vi "Parameter Set Write Single.vi"(8 "error in":errorcluster, 9 "Channel Index":i32, 10 "Parameter Set STS":i32, 11 "Parameter Set in":refnum<class "Parameter Set.lvclass">) -> (0 "error out":errorcluster, 3 "Parameter Set out":refnum<class "Parameter Set.lvclass">)   [LabVIEW 2023, in "Parameter Set.lvclass"]
uses:
  Parameter Set.lvclass
  <vilib>/ADAS Replay HIL/Channels/Tag Wrapper/Tag Wrapper.lvlib
  <vilib>/ADAS Replay HIL/Channels/Tag Wrapper/Polymorphic/Write Channel (I32).vi
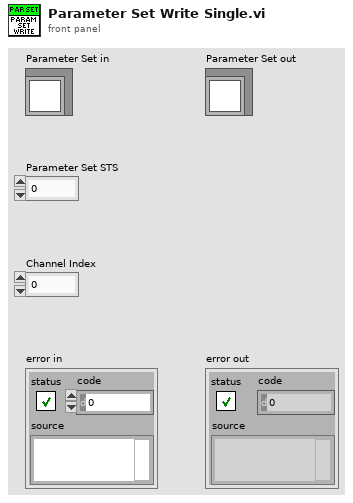
[diagram p1: front panel]
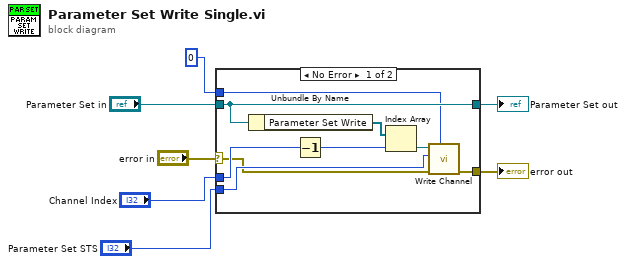
[diagram p0: block diagram]
diagram:
  n1 = case shown="No Error" "error in" {
    selector: "error in" -> [w11 w18]
    tunnel: [w10 w18] -> w6
    tunnel: [w9 w17] -> w4
    tunnel: "Parameter Set in" -> [w9 w17]
    tunnel: "Channel Index" -> [w13 _]
    tunnel: "Parameter Set STS" -> [w12 _]
    tunnel: 0 ("Timeout (ms)") -> [w8 _]
    frame No Error {
      n2 = Unbundle By Name(w9) -> ("Parameter Set Write"=w15:refnum<k21>[])
      n3 = Decrement(x=w13) -> (x-1=w16:i32)
      n4 = Index Array(array=w15, index=w16) -> (element=w14:refnum<k21>)
      n5 = call-poly <vilib>:"Write Channel.vi"("Timeout (ms)"=w8, "error in"=w11, "Value to Write"=w12, "ADAS HIL Channel in"=w14) -> ("error out"=w10:errorcluster)  [unwired: 5 in, 2 out]
    }
    frame Error {
    }
  }
  "error out" <- w6
  "Parameter Set out" <- w4
